vi "Autonomous Independent.vi"   [LabVIEW 2015]
doc: "This VI is called when autonomous begins, and will automatically be terminated when autonomous ends. You can carry out timed or sensor driven robot movement independently without needing to return to the caller."
uses:
  <vilib>/Rock Robotics/WPI/Utilities/WPI_GetSetVariantRefNum.vi
  <vilib>/Rock Robotics/Network Tables/NT Read String.vi
  <vilib>/Rock Robotics/Network Tables/NT Read Number.vi
  <vilib>/Rock Robotics/Network Tables/NT Read Boolean.vi
  <vilib>/Rock Robotics/Network Tables/NT Write Boolean.vi
  <vilib>/Rock Robotics/Network Tables/NT Write Numeric Array.vi
panel:
  # "Be sure to right-click and choose Data Operations>>Make Current Value default if you want to save the array values with the VI"
types:
  T1 = typedef "WPI_JoystickDevRef.ctl" = cluster{"Device":T2}
  T2 = typedef "WPI_JoystickDeviceEnum.ctl" = enum16{"USB 0", "USB 1", "USB 2", "USB 3", "USB 4", "USB 5"}
  T3 = typedef "WPI_MotorControlDeviceRef.ctl" = cluster{"DeviceStatus":errorcluster, "Type":T4, "PWM":cluster{"PWM Channel":T5, "DeadBand":T6}, "CAN":cluster{"Device Number":u8, "Control Mode":T7, "Semaphore":T8, "Max Vout":dbl, "TalonSRX Control Mode":T9}, "Invert":bool}
  T4 = typedef "WPI_MotorControlType.ctl" = enum16{"PWM", "CAN", "CANTalonSRX"}
  T5 = typedef "FPGA_DIOPWMChannel.ctl" = enum8{"PWM 0", "PWM 1", "PWM 2", "PWM 3", "PWM 4", "PWM 5", "PWM 6", "PWM 7", "PWM 8", "PWM 9", "PWM MXP 0", "PWM MXP 1", "PWM MXP 2", "PWM MXP 3", "PWM MXP 4", "PWM MXP 5", "PWM MXP 6", "PWM MXP 7", "PWM MXP 8", "PWM MXP 9", "Invalid"}
  T6 = typedef "WPI_PWMDeadband.ctl" = cluster{"Name":string, "maxPositivePwm":i32, "minPositivePwm":i32, "centerPwm":i32, "maxNegativePwm":i32, "minNegativePwm":i32, "angularRange":u16}
  T7 = typedef "WPI_CANJaguar_ControlMode.ctl" = enum8{"Percent VBus", "Current", "Speed", "Position", "Voltage"}
  T8 = typedef "Semaphore RefNum" = refnum<k1>
  T9 = typedef "WPI_CANTalonSRX_APIControlMode.ctl" = enum8{"Percent VBus", "Speed", "Position", "Slave", "Unchanged / Invalid", "Voltage Compensation", "Current", "Motion Profile"}
  T10 = typedef "WPI_RobotDriveDevRef.ctl" = cluster{"DevStatus":errorcluster, "Motors[]":T3[], "Square Inputs":bool, "Max Output":dbl}
  T11 = typedef "WPI_EncoderDevRef.ctl" = cluster{"DevStatus":errorcluster, "EncoderIndex":T12, "CounterIndex":T13, "DistancePerCount":dbl, "Decoding Type":T14}
  T12 = typedef "FPGA_EncoderIdx.ctl" = enum8{"Enc 0", "Enc 1", "Enc 2", "Enc 3", "Enc 4", "Enc 5", "Enc 6", "Enc 7", "Invalid"}
  T13 = typedef "FPGA_CounterCtrSystemIndex.ctl" = enum8{"Ctr 0", "Ctr 1", "Ctr 2", "Ctr 3", "Ctr 4", "Ctr 5", "Ctr 6", "Ctr 7", "Invalid"}
  T14 = typedef "WPI_EncoderType.ctl" = enum16{"1x", "2x", "4x"}
  T15 = typedef "WPI_GyroDevRef.ctl" = cluster{"DevStatus":errorcluster, "Analog Channel":T16, "Offset":dbl, "Gain (VoltsPerDegree/Second)":dbl, "Gyro Type":enum16{"Analog", "XRS450"}, "Handle":i32, "SPI Bus":T17, "Device Found":bool, "Sample Rate":dbl, "Calibrate On Open":bool}
  T16 = typedef "FPGA_AIChannel.ctl" = enum8{"AI 0", "AI 1", "AI 2", "AI 3", "AI MXP 0", "AI MXP 1", "AI MXP 2", "AI MXP 3", "Invalid"}
  T17 = typedef "spi_bus.ctl" = enum16{"SPI On-Board, CS0", "SPI On-Board, CS1", "SPI On-Board, CS2", "SPI On-Board, CS3", "SPI MXP", "Invalid"}
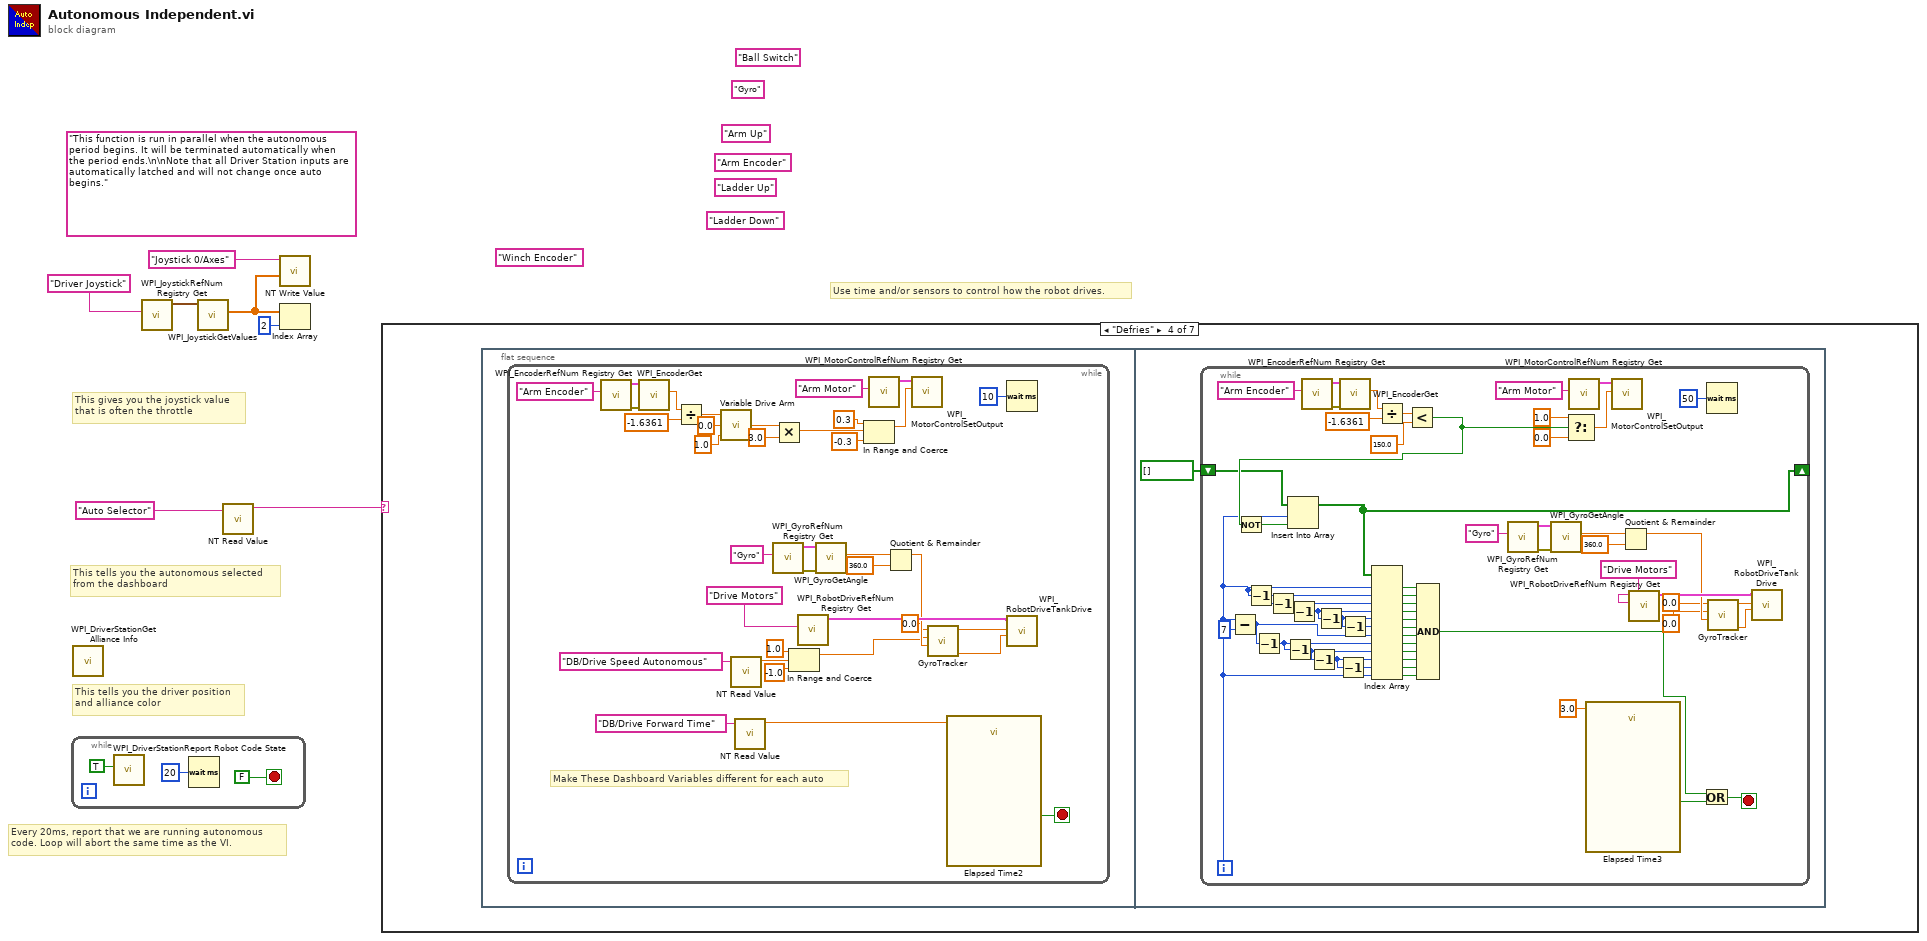
[diagram p0: block diagram]
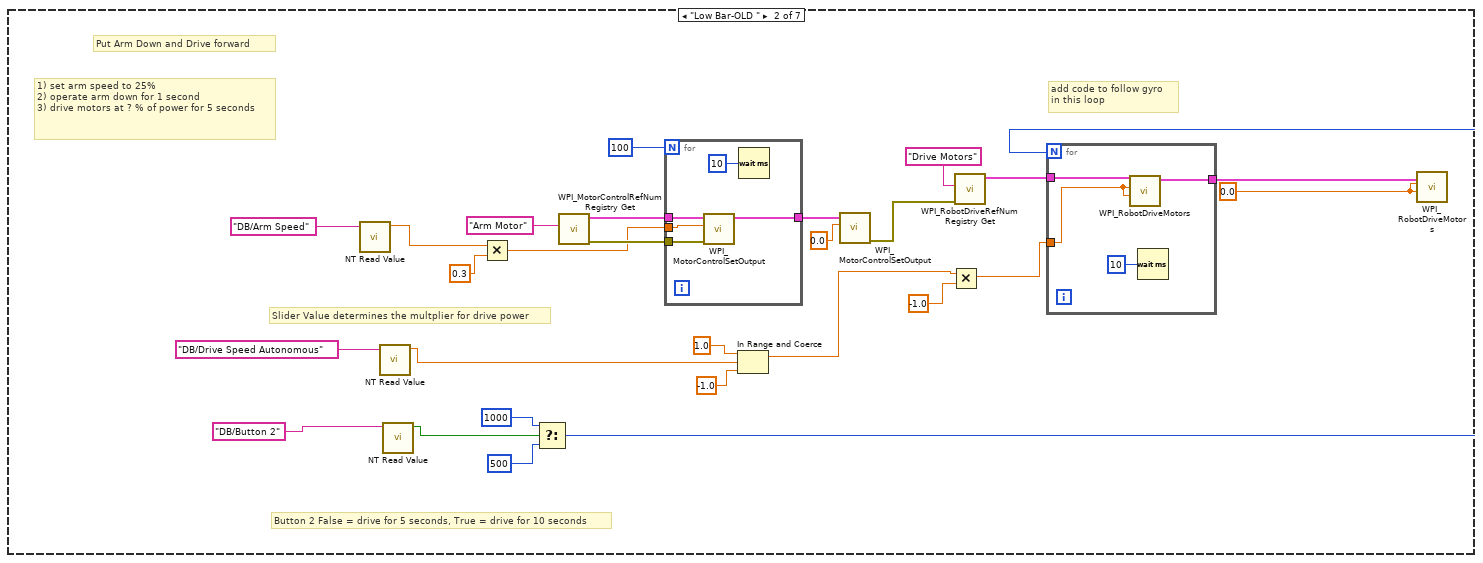
[diagram p3: hidden frame]
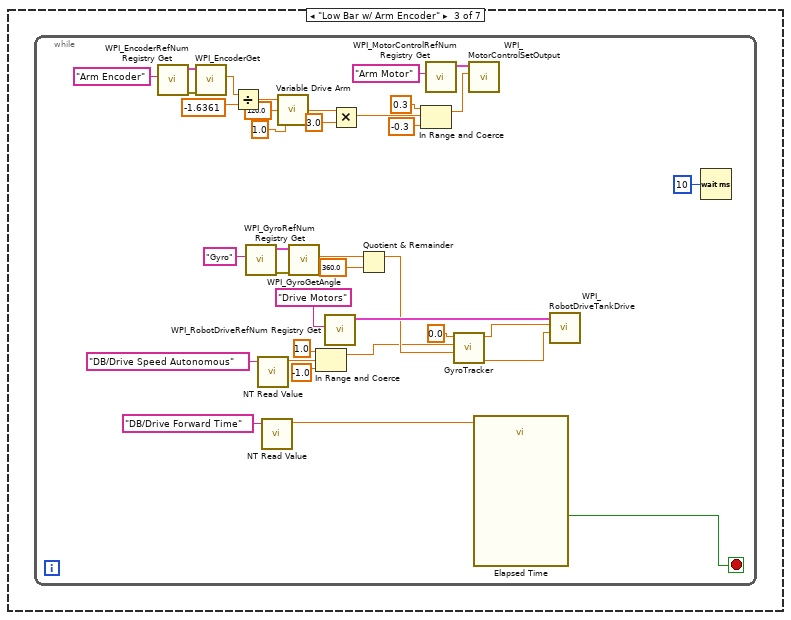
[diagram p4: hidden frame]
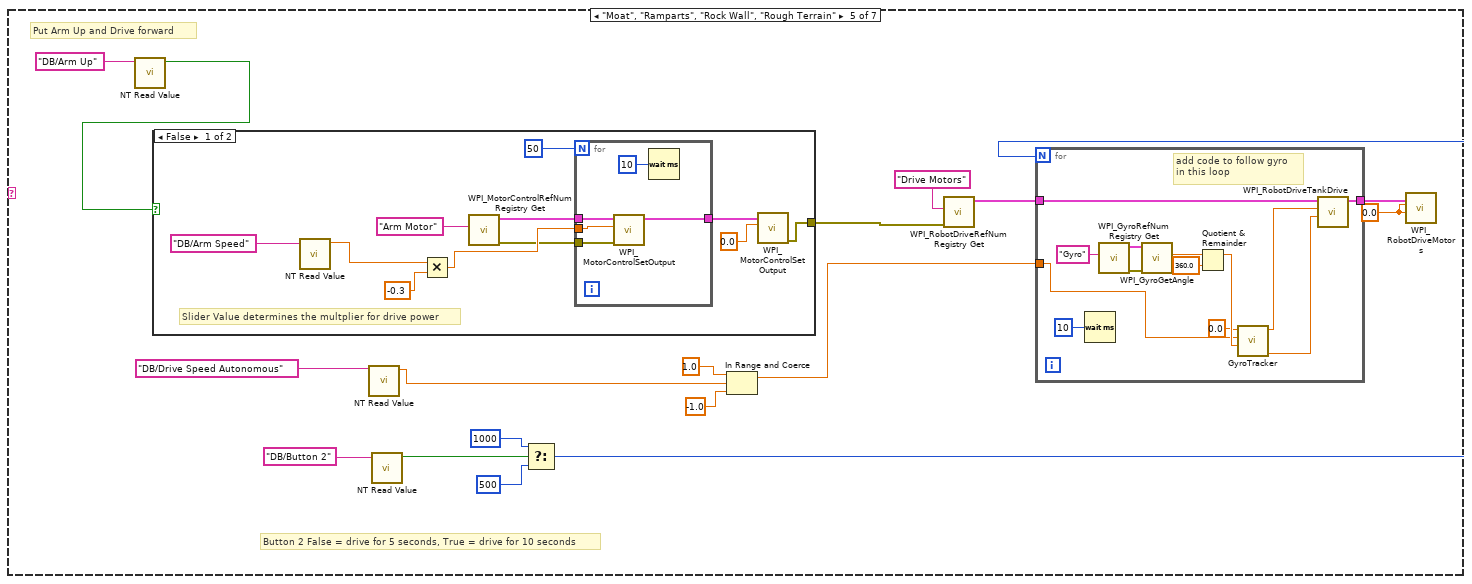
[diagram p5: hidden frame]
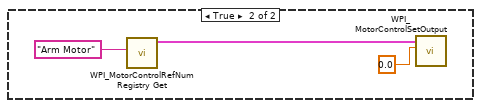
[diagram p6: hidden frame]
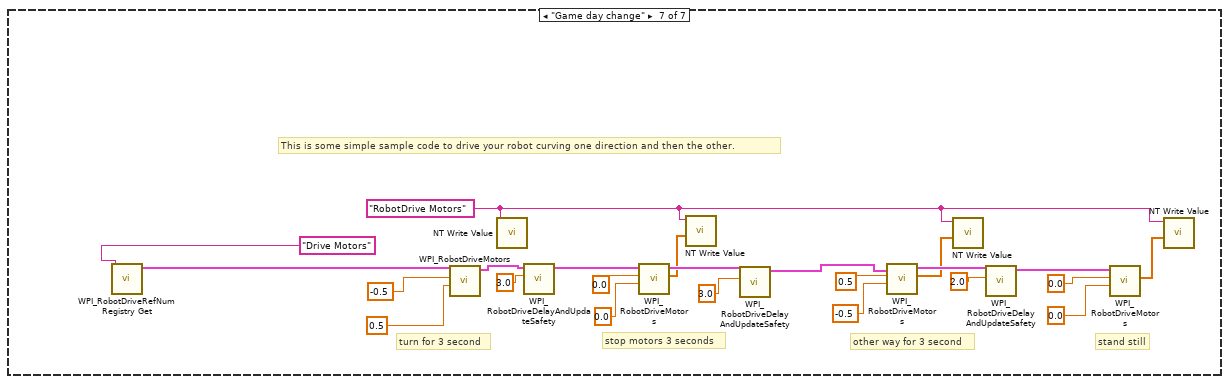
[diagram p8: hidden frame]
diagram:
  (unwired) "Arm Up" ("refnum name")
  (unwired) "Winch Encoder" ("refnum name")
  (unwired) "Ladder Down" ("refnum name")
  (unwired) "Ladder Up" ("refnum name")
  (unwired) "Arm Encoder" ("refnum name")
  (unwired) "Ball Switch" ("refnum name")
  (unwired) "Gyro" ("refnum name")
  (unwired) "This function is run in parallel when the autonomous period begins. It will be terminated automatically when the period ends.\n\nNote that all Driver Station inputs are automatically latched and will not change once auto begins."
  # "This tells you the autonomous selected\nfrom the dashboard"
  # "Every 20ms, report that we are running autonomous\ncode. Loop will abort the same time as the VI."
  # "This gives you the joystick value\nthat is often the throttle"
  # "Use time and/or sensors to control how the robot drives."
  # "This tells you the driver position\nand alliance color"
  n1 = while {
    stop <- FALSE stop-if-true
    n2 = call <vilib>:"WPI_DriverStationReport Robot Code State.vi"("Autonomous"=TRUE) -> ()  [unwired: 10 in, 1 out]
    n3 = Wait (ms)(milliseconds to wait=u32 20) -> ()  [unwired: 1 out]
  }
  n4 = call <vilib>:"WPI_DriverStationGet Alliance Info.vi"() -> ()  [unwired: 12 out]
  n5 = call <vilib>:"WPI_JoystickRefNum Registry Get.vi"("refnum name"="Driver Joystick") -> ("JoystickDevRef"=w6:T1)  [unwired: 1 in, 9 out]
  n6 = call <vilib>:"WPI_JoystickGetValues.vi"("JoystickDevRef"=w6) -> ("Axes"=w2:dbl[])  [unwired: 6 in, 4 out]
  n7 = call-poly <vilib>:"NT Read Value.vi"("Name"="Auto Selector") -> ("String"=w3:string)  [unwired: 9 in, 1 out]
  n8 = call-poly <vilib>:"NT Write Value.vi"("Numeric Array"=w2, "Name"="Joystick 0/Axes") -> ()  [unwired: 9 in, 1 out]
  n9 = Index Array(array=w2, index=2) -> ()  [unwired: 1 out]
  n10 = case shown="\"Defries\"" w3 {
    frame Default {
      # "You can put your main auto here, or you can right-click on the case and make any\nother frame be the default case."
      # "This is the frame that will execute if no selection is made, or if it is not recognized"
    }
    frame "Low Bar-OLD " {
      w23 = 0.0 ("Y axis value")
      # "Button 2 False = drive for 5 seconds, True = drive for 10 seconds"
      # "Slider Value determines the multplier for drive power"
      # "add code to follow gyro\nin this loop"
      # "1) set arm speed to 25%\n2) operate arm down for 1 second\n3) drive motors at ? % of power for 5 seconds"
      # "Put Arm Down and Drive forward"
      n11 = call-poly <vilib>:"NT Read Value.vi"("Name"="DB/Arm Speed") -> ("Numeric"=w35:dbl)  [unwired: 9 in, 1 out]
      n12 = call-poly <vilib>:"NT Read Value.vi"("Name"="DB/Drive Speed Autonomous") -> ("Numeric"=w19:dbl)  [unwired: 9 in, 1 out]
      n13 = call-poly <vilib>:"NT Read Value.vi"("Name"="DB/Button 2") -> ("Boolean"=w15:bool)  [unwired: 9 in, 1 out]
      n14 = Multiply(x=w35, y=0.3) -> (x*y=w30:dbl)
      n15 = Select(t=1000, s=w15, f=500) -> (s? t:f=w12:i32)
      n16 = call <vilib>:"WPI_MotorControlRefNum Registry Get.vi"("refnum name"="Arm Motor") -> ("error out"=w31:errorcluster, "MotorControlDevRef"=w32:T3)  [unwired: 9 in]
      n17 = for {
        N: 100 -> [_]
        tunnel: w32 -> [w45]
        tunnel: w31 -> [w44]
        tunnel: w30 -> [w43]
        tunnel: [w42] -> w29
        n18 = call <vilib>:"WPI_MotorControlSetOutput.vi"("error in (no error)"=w44, "Output"=w43, "MotorControlDevRef"=w45) -> ("MotorControlDevRef"=w42:T3)  [unwired: 6 in, 2 out]
        n19 = Wait (ms)(milliseconds to wait=u32 10) -> ()  [unwired: 1 out]
      }
      n20 = In Range and Coerce(upper limit=1.0, x=w19, lower limit=-1.0) -> (coerced(x)=w16:dbl)  [unwired: 1 out]
      n21 = call <vilib>:"WPI_MotorControlSetOutput.vi"("Output"=0.0, "MotorControlDevRef"=w29) -> ("error out"=w26:errorcluster)  [unwired: 7 in, 2 out]
      n22 = Multiply(x=w16, y=-1.0) -> (x*y=w21:dbl)
      n23 = call <vilib>:"WPI_RobotDriveRefNum Registry Get.vi"("error in (no error)"=w26, "refnum name"="Drive Motors") -> ("RobotDriveDevRef"=w25:T10)  [unwired: 9 out]
      n24 = for {
        N: w12 -> [_]
        tunnel: w25 -> [w41]
        tunnel: w21 -> [w40]
        tunnel: [w38] -> w24
        n25 = call <vilib>:"WPI_RobotDriveMotors.vi"("RightSpeed"=w40, "LeftSpeed"=w40, "RobotDriveDevRef"=w41) -> ("RobotDriveDevRef"=w38:T10)  [unwired: 6 in, 2 out]
        n26 = Wait (ms)(milliseconds to wait=u32 10) -> ()  [unwired: 1 out]
      }
      n27 = call <vilib>:"WPI_RobotDriveMotors.vi"("RightSpeed"=w23, "LeftSpeed"=w23, "RobotDriveDevRef"=w24) -> ()  [unwired: 6 in, 3 out]
    }
    frame "Low Bar w/ Arm Encoder" {
      n28 = while {
        stop <- w82 stop-if-true
        n29 = call <vilib>:"WPI_EncoderRefNum Registry Get.vi"("refnum name"="Arm Encoder") -> ("error out"=w75:errorcluster, "EncoderDevRef"=w76:T11)  [unwired: 9 in]
        n30 = call <vilib>:"WPI_EncoderGet.vi"("error in (no error)"=w75, "EncoderDevRef"=w76) -> ("Distance"=w77:dbl)  [unwired: 4 in, 5 out]
        n31 = Divide(x=w77, y=-1.6361 ("Arm Calibration")) -> (x/y=w74:dbl)
        n32 = call <vilib>:"WPI_GyroRefNum Registry Get.vi"("refnum name"="Gyro") -> ("error out"=w52:errorcluster, "GyroDevRef"=w53:T15)  [unwired: 9 in]
        n33 = call-poly <vilib>:"NT Read Value.vi"("Name"="DB/Drive Speed Autonomous") -> ("Numeric"=w60:dbl)  [unwired: 9 in, 1 out]
        n34 = call-poly <vilib>:"NT Read Value.vi"("Name"="DB/Drive Forward Time") -> ("Numeric"=w58:dbl)  [unwired: 9 in, 1 out]
        n35 = call "Variable Drive Arm.vi"("Max Speed"=1.0, "Wanted Angle"=120.0, "Encoder"=w74) -> ("Motor Controller"=w67:dbl)
        n36 = call <vilib>:"WPI_GyroGetAngle.vi"("error in"=w52, "GyroDevRef"=w53) -> ("Angle"=w55:dbl)  [unwired: 5 in, 4 out]
        n37 = In Range and Coerce(upper limit=1.0, x=w60, lower limit=-1.0) -> (coerced(x)=w49:dbl)  [unwired: 1 out]
        n38 = call <vilib>:"WPI_RobotDriveRefNum Registry Get.vi"("refnum name"="Drive Motors") -> ("RobotDriveDevRef"=w64:T10)  [unwired: 1 in, 9 out]
        n39 = Multiply(x=w67, y=3.0) -> (x*y=w65:dbl)
        n40 = Quotient & Remainder(x=w55, y=360.0) -> (x-y*floor(x/y)=w51:dbl)  [unwired: 1 out]
        n41 = In Range and Coerce(upper limit=0.3, x=w65, lower limit=-0.3) -> (coerced(x)=w70:dbl)  [unwired: 1 out]
        n42 = call <vilib>:"WPI_MotorControlRefNum Registry Get.vi"("refnum name"="Arm Motor") -> ("MotorControlDevRef"=w71:T3)  [unwired: 9 in, 1 out]
        n43 = call "GyroTracker.vi"("Gyro Angle"=w51, "Target Speed"=w49, "Target Direction (degrees)"=0.0) -> ("Right Wheel Speed"=w47:dbl, "Left Wheel Speed"=w48:dbl)  [unwired: 7 in]
        n44 = call <vilib>:"WPI_MotorControlSetOutput.vi"("Output"=w70, "MotorControlDevRef"=w71) -> ()  [unwired: 7 in, 3 out]
        n45 = call "Elapsed Time"("Time Target (s)"=w58) -> ("Time has Elapsed"=w82:bool)  [unwired: 11 in, 7 out]
        n46 = call <vilib>:"WPI_RobotDriveTankDrive.vi"("Right axis value"=w47, "Left axis value"=w48, "RobotDriveDevRef"=w64) -> ()  [unwired: 6 in, 3 out]
        n47 = Wait (ms)(milliseconds to wait=u32 10) -> ()  [unwired: 1 out]
      }
    }
    frame "Defries" {
      n48 = flat-sequence {
        frame #0 {
          n49 = while {
            stop <- w118 stop-if-true
            # "Make These Dashboard Variables different for each auto"
            n50 = call <vilib>:"WPI_EncoderRefNum Registry Get.vi"("refnum name"="Arm Encoder") -> ("error out"=w111:errorcluster, "EncoderDevRef"=w112:T11)  [unwired: 9 in]
            n51 = call <vilib>:"WPI_EncoderGet.vi"("error in (no error)"=w111, "EncoderDevRef"=w112) -> ("Distance"=w113:dbl)  [unwired: 4 in, 5 out]
            n52 = Divide(x=w113, y=-1.6361 ("Arm Calibration")) -> (x/y=w110:dbl)
            n53 = call "Variable Drive Arm.vi"("Max Speed"=1.0, "Wanted Angle"=0.0, "Encoder"=w110) -> ("Motor Controller"=w103:dbl)
            n54 = call-poly <vilib>:"NT Read Value.vi"("Name"="DB/Drive Speed Autonomous") -> ("Numeric"=w97:dbl)  [unwired: 9 in, 1 out]
            n55 = call-poly <vilib>:"NT Read Value.vi"("Name"="DB/Drive Forward Time") -> ("Numeric"=w95:dbl)  [unwired: 9 in, 1 out]
            n56 = call <vilib>:"WPI_GyroRefNum Registry Get.vi"("refnum name"="Gyro") -> ("error out"=w86:errorcluster, "GyroDevRef"=w87:T15)  [unwired: 9 in]
            n57 = Multiply(x=w103, y=3.0) -> (x*y=w101:dbl)
            n58 = In Range and Coerce(upper limit=1.0, x=w97, lower limit=-1.0) -> (coerced(x)=w83:dbl)  [unwired: 1 out]
            n59 = call <vilib>:"WPI_RobotDriveRefNum Registry Get.vi"("refnum name"="Drive Motors") -> ("RobotDriveDevRef"=w93:T10)  [unwired: 1 in, 9 out]
            n60 = call <vilib>:"WPI_GyroGetAngle.vi"("error in"=w86, "GyroDevRef"=w87) -> ("Angle"=w89:dbl)  [unwired: 5 in, 4 out]
            n61 = In Range and Coerce(upper limit=0.3, x=w101, lower limit=-0.3) -> (coerced(x)=w106:dbl)  [unwired: 1 out]
            n62 = call <vilib>:"WPI_MotorControlRefNum Registry Get.vi"("refnum name"="Arm Motor") -> ("MotorControlDevRef"=w107:T3)  [unwired: 9 in, 1 out]
            n63 = Quotient & Remainder(x=w89, y=360.0) -> (x-y*floor(x/y)=w85:dbl)  [unwired: 1 out]
            n64 = call <vilib>:"WPI_MotorControlSetOutput.vi"("Output"=w106, "MotorControlDevRef"=w107) -> ()  [unwired: 7 in, 3 out]
            n65 = call "GyroTracker.vi"("Gyro Angle"=w85, "Target Speed"=w83, "Target Direction (degrees)"=0.0) -> ("Right Wheel Speed"=w91:dbl, "Left Wheel Speed"=w92:dbl)  [unwired: 7 in]
            n66 = call "Elapsed Time2"("Time Target (s)"=w95) -> ("Time has Elapsed"=w118:bool)  [unwired: 11 in, 7 out]
            n67 = Wait (ms)(milliseconds to wait=u32 10) -> ()  [unwired: 1 out]
            n68 = call <vilib>:"WPI_RobotDriveTankDrive.vi"("Right axis value"=w91, "Left axis value"=w92, "RobotDriveDevRef"=w93) -> ()  [unwired: 6 in, 3 out]
          }
        }
        frame #1 {
          n69 = while {
            shift-right: [w124] -> _
            shift-left: bool[] [] -> [w125]
            i -> [w123]
            stop <- w128 stop-if-true
            n70 = Subtract(x=w123, y=7) -> (x-y=w145:i32)
            n71 = Decrement(x=w123) -> (x-1=w148:i32)
            n72 = Decrement(x=w145) -> (x-1=w144:i32)
            n73 = Decrement(x=w148) -> (x-1=w150:i32)
            n74 = Decrement(x=w144) -> (x-1=w143:i32)
            n75 = Decrement(x=w150) -> (x-1=w152:i32)
            n76 = call <vilib>:"WPI_EncoderRefNum Registry Get.vi"("refnum name"="Arm Encoder") -> ("error out"=w158:errorcluster, "EncoderDevRef"=w159:T11)  [unwired: 9 in]
            n77 = Decrement(x=w143) -> (x-1=w141:i32)
            n78 = Decrement(x=w152) -> (x-1=w149:i32)
            n79 = Decrement(x=w141) -> (x-1=w142:i32)
            n80 = call <vilib>:"WPI_EncoderGet.vi"("error in (no error)"=w158, "EncoderDevRef"=w159) -> ("Distance"=w160:dbl)  [unwired: 4 in, 5 out]
            n81 = Decrement(x=w149) -> (x-1=w151:i32)
            n82 = Divide(x=w160, y=-1.6361 ("Arm Calibration")) -> (x/y=w153:dbl)
            n83 = Less?(x=w153, y=150.0) -> (x < y?=w126:bool)
            n84 = Not(x=w126) -> (.not. x?=w120:bool)
            n85 = Insert Into Array(array=w125, index=w123, new element=w120) -> (w124:bool[])
            n86 = Index Array(array=w124, index #1=w123, index #2=w148, index #3=w150, index #4=w152, index #5=w149, index #6=w151, index #7=w145, index #8=w144, index #9=w143, index #10=w141, index #11=w142, index #12=w123) -> (element #1=w140:bool, element #2=w139:bool, element #3=w138:bool, element #4=w137:bool, element #5=w136:bool, element #6=w135:bool, element #7=w134:bool, element #8=w133:bool, element #9=w132:bool, element #10=w131:bool, element #11=w130:bool, element #12=w122:bool)
            n87 = Compound Arithmetic op=AND(w140, w139, w138, w137, w136, w135, w134, w133, w132, w131, w130, w122) -> (w121:bool)
            n88 = call <vilib>:"WPI_GyroRefNum Registry Get.vi"("refnum name"="Gyro") -> ("error out"=w166:errorcluster, "GyroDevRef"=w167:T15)  [unwired: 9 in]
            n89 = call <vilib>:"WPI_GyroGetAngle.vi"("error in"=w166, "GyroDevRef"=w167) -> ("Angle"=w169:dbl)  [unwired: 5 in, 4 out]
            n90 = Select(t=1.0, s=w126, f=0.0) -> (s? t:f=w156:dbl)
            n91 = call <vilib>:"WPI_MotorControlRefNum Registry Get.vi"("refnum name"="Arm Motor") -> ("MotorControlDevRef"=w175:T3)  [unwired: 9 in, 1 out]
            n92 = call "Elapsed Time3"("Time Target (s)"=3.0) -> ("Time has Elapsed"=w129:bool)  [unwired: 11 in, 7 out]
            n93 = call <vilib>:"WPI_MotorControlSetOutput.vi"("Output"=w156, "MotorControlDevRef"=w175) -> ()  [unwired: 7 in, 3 out]
            n94 = Quotient & Remainder(x=w169, y=360.0) -> (x-y*floor(x/y)=w165:dbl)  [unwired: 1 out]
            n95 = call <vilib>:"WPI_RobotDriveRefNum Registry Get.vi"("refnum name"="Drive Motors") -> ("RobotDriveDevRef"=w172:T10)  [unwired: 1 in, 9 out]
            n96 = Or(x=w121, y=w129) -> (x .or. y?=w128:bool)
            n97 = Wait (ms)(milliseconds to wait=u32 50) -> ()  [unwired: 1 out]
            n98 = call "GyroTracker.vi"("Gyro Angle"=w165, "Target Speed"=0.0, "Target Direction (degrees)"=0.0) -> ("Right Wheel Speed"=w147:dbl, "Left Wheel Speed"=w171:dbl)  [unwired: 7 in]
            n99 = call <vilib>:"WPI_RobotDriveTankDrive.vi"("Right axis value"=w147, "Left axis value"=w171, "RobotDriveDevRef"=w172) -> ()  [unwired: 6 in, 3 out]
          }
        }
      }
    }
    frame "Moat", "Ramparts", "Rock Wall", "Rough Terrain" {
      w190 = 0.0 ("Y axis value")
      # "Button 2 False = drive for 5 seconds, True = drive for 10 seconds"
      # "Put Arm Up and Drive forward"
      n100 = call-poly <vilib>:"NT Read Value.vi"("Name"="DB/Arm Up") -> ("Boolean"=w178:bool)  [unwired: 9 in, 1 out]
      n101 = case shown="False" w178 {
        tunnel: [w194 _] -> w179
        frame False {
          # "Slider Value determines the multplier for drive power"
          n102 = call-poly <vilib>:"NT Read Value.vi"("Name"="DB/Arm Speed") -> ("Numeric"=w199:dbl)  [unwired: 9 in, 1 out]
          n103 = Multiply(x=w199, y=-0.3) -> (x*y=w204:dbl)
          n104 = call <vilib>:"WPI_MotorControlRefNum Registry Get.vi"("refnum name"="Arm Motor") -> ("error out"=w203:errorcluster, "MotorControlDevRef"=w202:T3)  [unwired: 9 in]
          n105 = for {
            N: 50 -> [_]
            tunnel: w202 -> [w208]
            tunnel: w203 -> [w207]
            tunnel: w204 -> [w206]
            tunnel: [w205] -> w195
            n106 = call <vilib>:"WPI_MotorControlSetOutput.vi"("error in (no error)"=w207, "Output"=w206, "MotorControlDevRef"=w208) -> ("MotorControlDevRef"=w205:T3)  [unwired: 6 in, 2 out]
            n107 = Wait (ms)(milliseconds to wait=u32 10) -> ()  [unwired: 1 out]
          }
          n108 = call <vilib>:"WPI_MotorControlSetOutput.vi"("Output"=0.0, "MotorControlDevRef"=w195) -> ("error out"=w194:errorcluster)  [unwired: 7 in, 2 out]
        }
        frame True {
          n109 = call <vilib>:"WPI_MotorControlRefNum Registry Get.vi"("refnum name"="Arm Motor") -> ("MotorControlDevRef"=w211:T3)  [unwired: 9 in, 1 out]
          n110 = call <vilib>:"WPI_MotorControlSetOutput.vi"("Output"=0.0, "MotorControlDevRef"=w211) -> ()  [unwired: 7 in, 3 out]
        }
      }
      n111 = call-poly <vilib>:"NT Read Value.vi"("Name"="DB/Drive Speed Autonomous") -> ("Numeric"=w188:dbl)  [unwired: 9 in, 1 out]
      n112 = call-poly <vilib>:"NT Read Value.vi"("Name"="DB/Button 2") -> ("Boolean"=w184:bool)  [unwired: 9 in, 1 out]
      n113 = Select(t=1000, s=w184, f=500) -> (s? t:f=w181:i32)
      n114 = In Range and Coerce(upper limit=1.0, x=w188, lower limit=-1.0) -> (coerced(x)=w177:dbl)  [unwired: 1 out]
      n115 = call <vilib>:"WPI_RobotDriveRefNum Registry Get.vi"("error in (no error)"=w179, "refnum name"="Drive Motors") -> ("RobotDriveDevRef"=w192:T10)  [unwired: 9 out]
      n116 = for {
        N: w181 -> [_]
        tunnel: w192 -> [w215]
        tunnel: w177 -> [w213]
        tunnel: [w214] -> w191
        # "add code to follow gyro\nin this loop"
        n117 = Wait (ms)(milliseconds to wait=u32 10) -> ()  [unwired: 1 out]
        n118 = call <vilib>:"WPI_GyroRefNum Registry Get.vi"("refnum name"="Gyro") -> ("error out"=w218:errorcluster, "GyroDevRef"=w219:T15)  [unwired: 9 in]
        n119 = call <vilib>:"WPI_GyroGetAngle.vi"("error in"=w218, "GyroDevRef"=w219) -> ("Angle"=w221:dbl)  [unwired: 5 in, 4 out]
        n120 = Quotient & Remainder(x=w221, y=360.0) -> (x-y*floor(x/y)=w217:dbl)  [unwired: 1 out]
        n121 = call "GyroTracker.vi"("Gyro Angle"=w217, "Target Speed"=w213, "Target Direction (degrees)"=0.0) -> ("Right Wheel Speed"=w223:dbl, "Left Wheel Speed"=w224:dbl)  [unwired: 7 in]
        n122 = call <vilib>:"WPI_RobotDriveTankDrive.vi"("Right axis value"=w223, "Left axis value"=w224, "RobotDriveDevRef"=w215) -> ("RobotDriveDevRef"=w214:T10)  [unwired: 6 in, 2 out]
      }
      n123 = call <vilib>:"WPI_RobotDriveMotors.vi"("RightSpeed"=w190, "LeftSpeed"=w190, "RobotDriveDevRef"=w191) -> ()  [unwired: 6 in, 3 out]
    }
    frame "Portcullis" {
    }
    frame "Game day change" {
      w230 = "RobotDrive Motors" ("Name")
      # "stop motors 3 seconds"
      # "This is some simple sample code to drive your robot curving one direction and then the other."
      # "stand still"
      # "other way for 3 second"
      # "turn for 3 second"
      n124 = call <vilib>:"WPI_RobotDriveRefNum Registry Get.vi"("refnum name"="Drive Motors") -> ("RobotDriveDevRef"=w227:T10)  [unwired: 1 in, 9 out]
      n125 = call <vilib>:"WPI_RobotDriveMotors.vi"("RightSpeed"=0.5 ("X axis value"), "LeftSpeed"=-0.5 ("X axis value"), "RobotDriveDevRef"=w227) -> ("RobotDriveDevRef"=w226:T10)  [unwired: 6 in, 2 out]
      n126 = call-poly <vilib>:"NT Write Value.vi"("Name"=w230) -> ()  [unwired: 10 in, 1 out]
      n127 = call <vilib>:"WPI_RobotDriveDelayAndUpdateSafety.vi"("Delay (s)"=3.0, "RobotDriveDevRef"=w226) -> ("RobotDriveDevRef 2"=w235:T10)  [unwired: 8 in, 1 out]
      n128 = call <vilib>:"WPI_RobotDriveMotors.vi"("RightSpeed"=0.0 ("X axis value"), "LeftSpeed"=0.0 ("X axis value"), "RobotDriveDevRef"=w235) -> ("Motor Values"=w231:dbl[], "RobotDriveDevRef"=w234:T10)  [unwired: 6 in, 1 out]
      n129 = call-poly <vilib>:"NT Write Value.vi"("Numeric Array"=w231, "Name"=w230) -> ()  [unwired: 9 in, 1 out]
      n130 = call <vilib>:"WPI_RobotDriveDelayAndUpdateSafety.vi"("Delay (s)"=3.0, "RobotDriveDevRef"=w234) -> ("RobotDriveDevRef 2"=w232:T10)  [unwired: 8 in, 1 out]
      n131 = call <vilib>:"WPI_RobotDriveMotors.vi"("RightSpeed"=-0.5 ("X axis value"), "LeftSpeed"=0.5 ("X axis value"), "RobotDriveDevRef"=w232) -> ("Motor Values"=w238:dbl[], "RobotDriveDevRef"=w244:T10)  [unwired: 6 in, 1 out]
      n132 = call-poly <vilib>:"NT Write Value.vi"("Numeric Array"=w238, "Name"=w230) -> ()  [unwired: 9 in, 1 out]
      n133 = call <vilib>:"WPI_RobotDriveDelayAndUpdateSafety.vi"("Delay (s)"=2.0, "RobotDriveDevRef"=w244) -> ("RobotDriveDevRef 2"=w245:T10)  [unwired: 8 in, 1 out]
      n134 = call <vilib>:"WPI_RobotDriveMotors.vi"("RightSpeed"=0.0 ("X axis value"), "LeftSpeed"=0.0 ("X axis value"), "RobotDriveDevRef"=w245) -> ("Motor Values"=w239:dbl[])  [unwired: 6 in, 2 out]
      n135 = call-poly <vilib>:"NT Write Value.vi"("Numeric Array"=w239, "Name"=w230) -> ()  [unwired: 9 in, 1 out]
    }
  }
